vi "OutProc.vi"(9 "Servos":cluster{T1[]}, 10 "ActuatorInputs":T9, 11 "Motors":cluster{T4[]}) -> ()   [LabVIEW 2015]
uses:
  Typedefs/ActuatorInputs.ctl
  <vilib>/Rock Robotics/WPI/MotorControl/WPI_MotorControlDeviceRef.ctl
  <vilib>/Rock Robotics/WPI/MotorControl/WPI_MotorControlType.ctl
  <vilib>/Rock Robotics/SystemInterfaces/DIO/FPGA_DIOPWMChannel.ctl
  <vilib>/Rock Robotics/WPI/PWM/WPI_PWMDeadband.ctl
  <vilib>/Rock Robotics/WPI/CAN/Jaguar/SubVIs/WPI_CANJaguar_ControlMode.ctl
  <vilib>/Rock Robotics/WPI/CAN/TalonSRX/WPI_CANTalonSRX_APIControlMode.ctl
  <vilib>/Rock Robotics/WPI/PWM/Servo/WPI_ServoDeviceRef.ctl
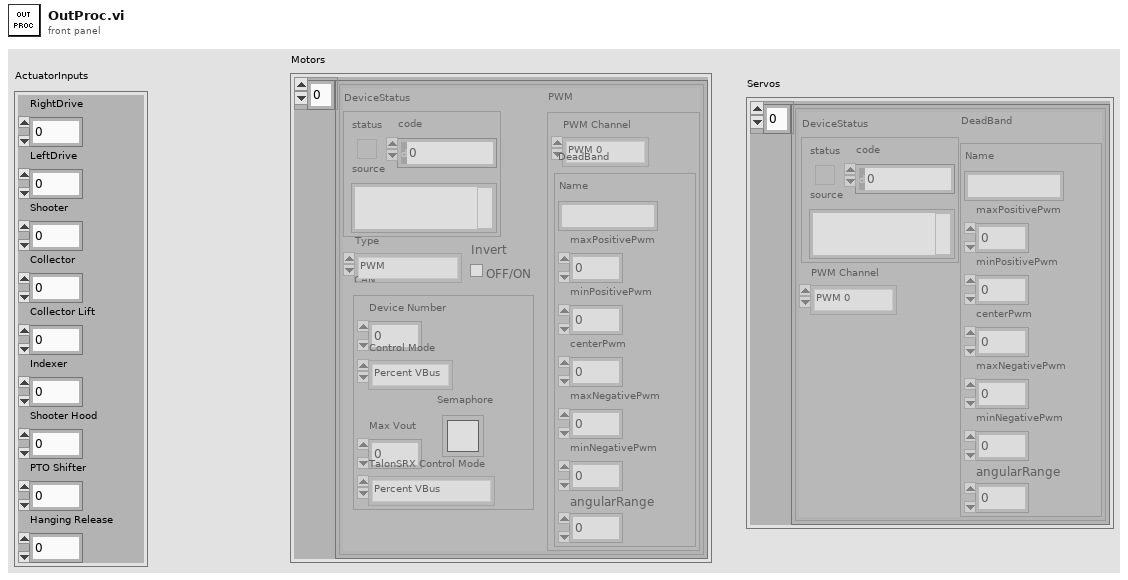
[diagram p1: front panel]
types:
  T1 = typedef "WPI_ServoDeviceRef.ctl" = cluster{"DeviceStatus":errorcluster, "PWM Channel":T2, "DeadBand":T3}
  T2 = typedef "FPGA_DIOPWMChannel.ctl" = enum8{"PWM 0", "PWM 1", "PWM 2", "PWM 3", "PWM 4", "PWM 5", "PWM 6", "PWM 7", "PWM 8", "PWM 9", "PWM MXP 0", "PWM MXP 1", "PWM MXP 2", "PWM MXP 3", "PWM MXP 4", "PWM MXP 5", "PWM MXP 6", "PWM MXP 7", "PWM MXP 8", "PWM MXP 9", "Invalid"}
  T3 = typedef "WPI_PWMDeadband.ctl" = cluster{"Name":string, "maxPositivePwm":i32, "minPositivePwm":i32, "centerPwm":i32, "maxNegativePwm":i32, "minNegativePwm":i32, "angularRange":u16}
  T4 = typedef "WPI_MotorControlDeviceRef.ctl" = cluster{"DeviceStatus":errorcluster, "Type":T5, "PWM":cluster{"PWM Channel":T2, "DeadBand":T3}, "CAN":cluster{"Device Number":u8, "Control Mode":T6, "Semaphore":T7, "Max Vout":dbl, "TalonSRX Control Mode":T8}, "Invert":bool}
  T5 = typedef "WPI_MotorControlType.ctl" = enum16{"PWM", "CAN", "CANTalonSRX"}
  T6 = typedef "WPI_CANJaguar_ControlMode.ctl" = enum8{"Percent VBus", "Current", "Speed", "Position", "Voltage"}
  T7 = typedef "Semaphore RefNum" = refnum<k1>
  T8 = typedef "WPI_CANTalonSRX_APIControlMode.ctl" = enum8{"Percent VBus", "Speed", "Position", "Slave", "Unchanged / Invalid", "Voltage Compensation", "Current", "Motion Profile"}
  T9 = typedef "ActuatorInputs.ctl" = cluster{"RightDrive":dbl, "LeftDrive":dbl, "Shooter":dbl, "Collector":dbl, "Collector Lift":dbl, "Indexer":dbl, "Shooter Hood":dbl, "PTO Shifter":dbl, "Hanging Release":dbl}
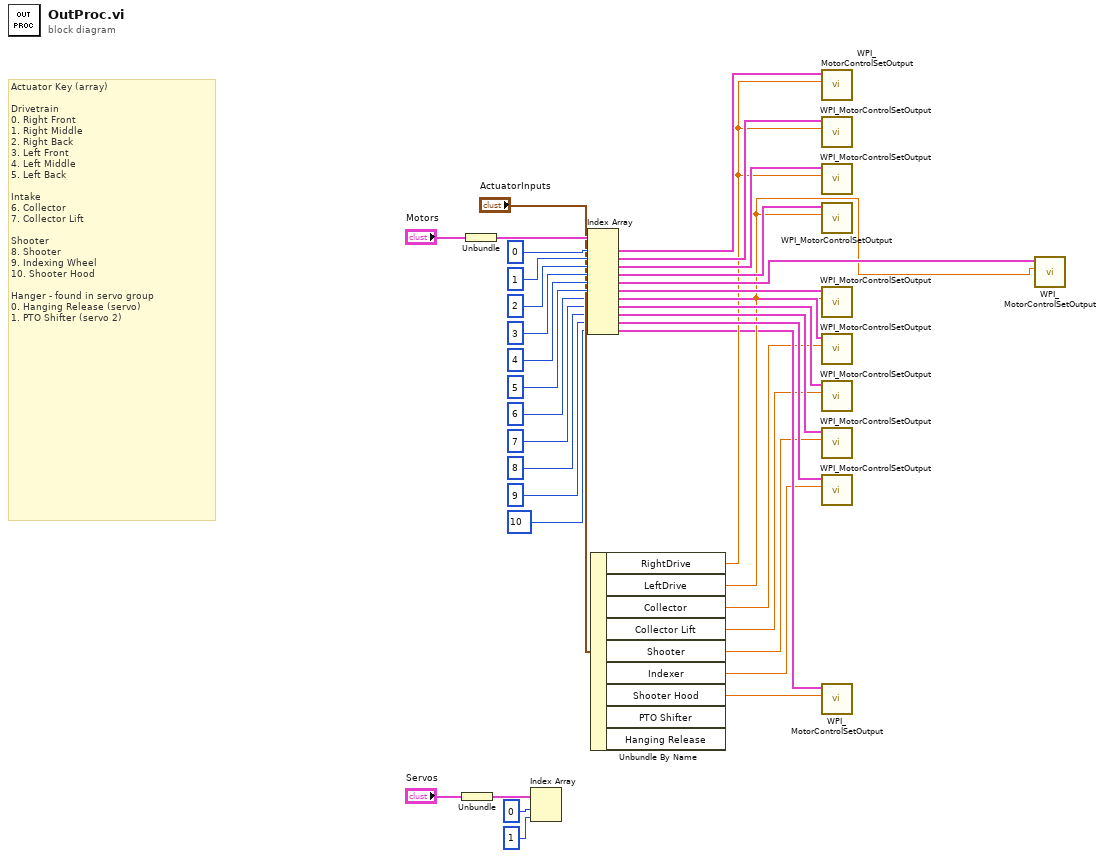
[diagram p0: block diagram]
diagram:
  # "Actuator Key (array)\n \nDrivetrain\n0. Right Front\n1. Right Middle\n2. Right Back\n3. Left Front\n4. Left Middle\n5. Left Back\n\nIntake\n6. Collector\n7. Collector Lift\n\nShooter\n8. Shooter\n9. Indexing Wheel\n10. Shooter Hood\n\nHanger - found in servo group\n0. Hanging Release (servo)\n1. PTO Shifter (servo 2)"
  n1 = Unbundle("Servos") -> (w6:T1[])
  n2 = Unbundle("Motors") -> (w36:T4[])
  n3 = Index Array(array=w6, index #1=0, index #2=1) -> ()  [unwired: 2 out]
  n4 = Index Array(array=w36, index #1=0, index #2=1, index #3=2, index #4=3, index #5=4, index #6=5, index #7=6, index #8=7, index #9=8, index #10=9, index #11=10) -> (element #1=w29:T4, element #2=w28:T4, element #3=w27:T4, element #4=w26:T4, element #5=w25:T4, element #6=w24:T4, element #7=w18:T4, element #8=w17:T4, element #9=w16:T4, element #10=w15:T4, element #11=w11:T4)
  n5 = Unbundle By Name("ActuatorInputs") -> ("RightDrive"=w14:dbl, "LeftDrive"=w13:dbl, "Collector"=w10:dbl, "Collector Lift"=w9:dbl, "Shooter"=w3:dbl, "Indexer"=w2:dbl, "Shooter Hood"=w1:dbl)  [unwired: 2 out]
  n6 = call <vilib>:"WPI_MotorControlSetOutput.vi"("Output"=w14, "MotorControlDevRef"=w29) -> ()  [unwired: 7 in, 3 out]
  n7 = call <vilib>:"WPI_MotorControlSetOutput.vi"("Output"=w14, "MotorControlDevRef"=w28) -> ()  [unwired: 7 in, 3 out]
  n8 = call <vilib>:"WPI_MotorControlSetOutput.vi"("Output"=w14, "MotorControlDevRef"=w27) -> ()  [unwired: 7 in, 3 out]
  n9 = call <vilib>:"WPI_MotorControlSetOutput.vi"("Output"=w13, "MotorControlDevRef"=w26) -> ()  [unwired: 7 in, 3 out]
  n10 = call <vilib>:"WPI_MotorControlSetOutput.vi"("Output"=w13, "MotorControlDevRef"=w24) -> ()  [unwired: 7 in, 3 out]
  n11 = call <vilib>:"WPI_MotorControlSetOutput.vi"("Output"=w10, "MotorControlDevRef"=w18) -> ()  [unwired: 7 in, 3 out]
  n12 = call <vilib>:"WPI_MotorControlSetOutput.vi"("Output"=w9, "MotorControlDevRef"=w17) -> ()  [unwired: 7 in, 3 out]
  n13 = call <vilib>:"WPI_MotorControlSetOutput.vi"("Output"=w3, "MotorControlDevRef"=w16) -> ()  [unwired: 7 in, 3 out]
  n14 = call <vilib>:"WPI_MotorControlSetOutput.vi"("Output"=w2, "MotorControlDevRef"=w15) -> ()  [unwired: 7 in, 3 out]
  n15 = call <vilib>:"WPI_MotorControlSetOutput.vi"("Output"=w1, "MotorControlDevRef"=w11) -> ()  [unwired: 7 in, 3 out]
  n16 = call <vilib>:"WPI_MotorControlSetOutput.vi"("Output"=w13, "MotorControlDevRef"=w25) -> ()  [unwired: 7 in, 3 out]
